vi "Invert Transformation Matrix.vi"(1 "4x4 Transformation Matrix":T1) -> (0 "Inverted 4x4 Transformation Matrix":T1)   [LabVIEW 2020, in "ar.lvlib"]
doc: "Invert a 4x4 Transformation Matrix using the fast method which relies on the symetrical properties of the rotation matrix."
uses:
  ar.lvlib
  <vilib>/Analysis/Matrix/Datatypes/RealMatrix.ctl
  <vilib>/Analysis/baseanly.llb/Real A x B.vi
  <vilib>/Analysis/NI_AALBase.lvlib
  <vilib>/Analysis/Matrix/NI_Matrix.lvlib
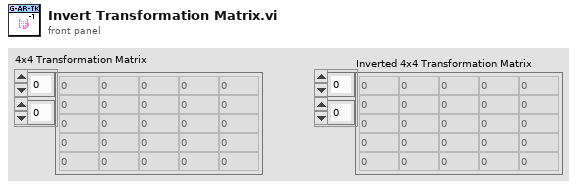
[diagram p1: front panel]
types:
  T1 = typedef "NI_Matrix.lvlib/RealMatrix.ctl" = dbl[][]
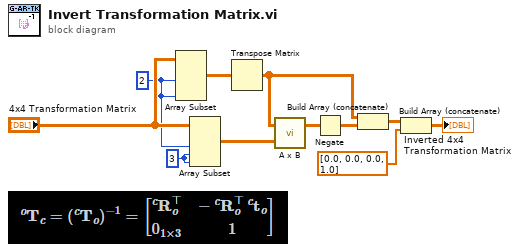
[diagram p0: block diagram]
diagram:
  w8 = 3 ("column N")
  w9 = 2 ("row N")
  n1 = Array Subset(array="4x4 Transformation Matrix", length (row)=w9, length (col)=w9) -> (w11:T1)  [unwired: 2 in]
  n2 = Array Subset(array="4x4 Transformation Matrix", length (row)=w9, index (col)=w8, length (col)=w8) -> (w7:T1)  [unwired: 1 in]
  n3 = Transpose Matrix(1:w11) -> (0:w6:T1)
  n4 = call-poly <vilib>:"A x B.vi"("B"=w7, "A"=w6) -> ("A x B"=w5:T1)  [unwired: 1 out]
  n5 = Negate(x=w5) -> (-x=w1:T1)
  n6 = Build Array (concatenate)(w6, w1) -> (w3:T1)
  n7 = Build Array (concatenate)(w3, dbl[] [0.0, 0.0, 0.0, 1.0]) -> (→"Inverted 4x4 Transformation Matrix":T1)
